vi "CSC_InitCableLocation.vi"(8 "error in (no error)":errorcluster, 11 "C-Alex in":refnum<class "CableSerialChain.lvclass">) -> (0 "error out":errorcluster, 3 "C-Alex out":refnum<class "CableSerialChain.lvclass">)   [LabVIEW 2014]
uses:
  Body/PointOnBody.ctl
  Body/Bodies.lvclass
  Cable.ctl
  CableSerialChain.lvclass
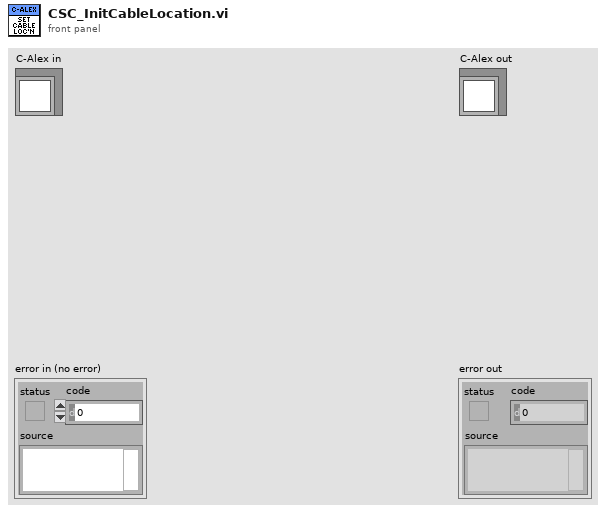
[diagram p1: front panel]
types:
  T1 = typedef "CableSerialChain.lvclass/Cable.ctl" = cluster{"RoutingPtsInLegCoSys":T2[], "Cable ID":i32}
  T2 = typedef "Bodies.lvclass/PointOnBody.ctl" = cluster{"Coord4":dbl[], "ID":i32}
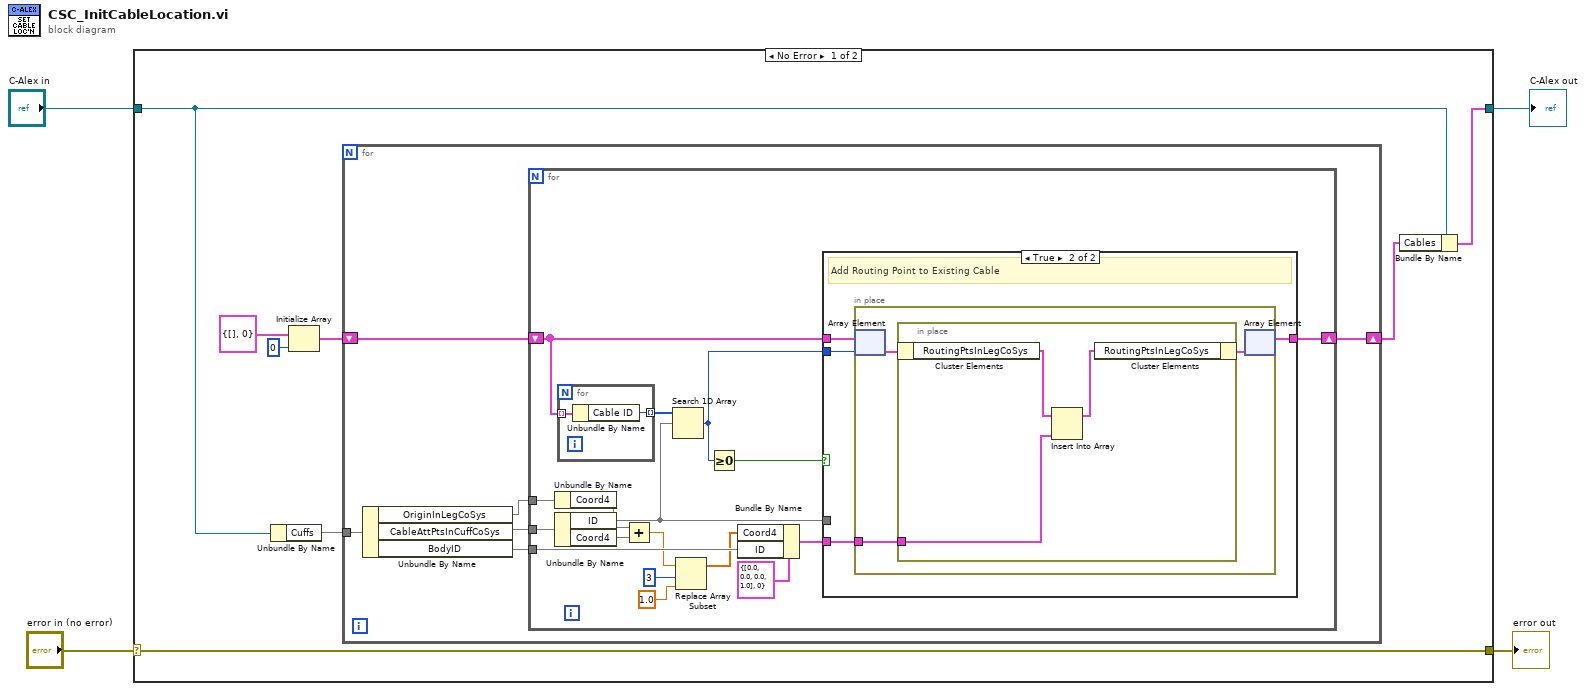
[diagram p0: block diagram]
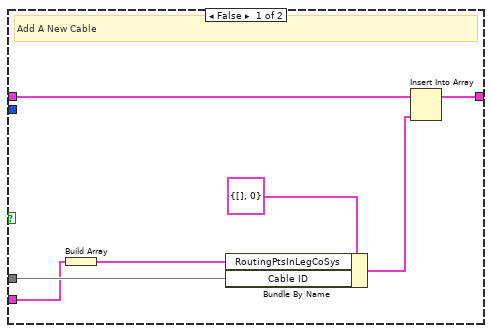
[diagram p2: hidden frame]
diagram:
  n1 = case shown="No Error" "error in (no error)" {
    selector: "error in (no error)" -> [w12 w56]
    tunnel: [w12 w56] -> w3
    tunnel: [w5 w55] -> w1
    tunnel: "C-Alex in" -> [w10 w55]
    frame No Error {
      n2 = Unbundle By Name(w10) -> ("Cuffs"=w11)
      n3 = Initialize Array(T1 {"RoutingPtsInLegCoSys"=[], "Cable ID"=0} ("Cable"), 0 ("dimension size")) -> (w9:T1[])
      n4 = for {
        tunnel: w11 -> [w18]
        shift-right: [w14] -> w6
        shift-left: w9 -> [w15]
        n5 = Unbundle By Name(w18) -> ("OriginInLegCoSys"=w13, "CableAttPtsInCuffCoSys"=w17, "BodyID"=w16)
        n6 = for {
          tunnel: w17 -> [w35]
          tunnel: w16 -> [w33]
          shift-right: [w28] -> w14
          shift-left: w15 -> [w26]
          tunnel: w13 -> [w25]
          n7 = Unbundle By Name(w25) -> ("Coord4"=w23)
          n8 = Unbundle By Name(w35) -> ("ID"=w27, "Coord4"=w24)
          n9 = for {
            tunnel: w26 -> [w54] mode=indexing
            tunnel: [w53] -> w32 mode=indexing
            n10 = Unbundle By Name(w54) -> ("Cable ID"=w53:i32)
          }
          n11 = Add(x=w23, y=w24) -> (x+y=w22:dbl)
          n12 = Search 1D Array(1D array=w32, element=w27) -> (index of element=w30:i32)  [unwired: 1 in]
          n13 = Replace Array Subset(array=w22, new element=1.0 ("new element/subarray"), index=3) -> (w21:dbl[])
          n14 = Greater Or Equal To 0?(x=w30) -> (x >= 0?=w31:bool)
          n15 = Bundle By Name(cluster=T2 {"Coord4"=[0.0, 0.0, 0.0, 1.0], "ID"=0} ("Point"), "Coord4"=w21, "ID"=w33) -> (w29:T2)
          n16 = case shown="True" w31 {
            tunnel: w30 -> [_ w45]
            tunnel: w26 -> [w42 w46]
            tunnel: w29 -> [w37 w43]
            tunnel: [w39 w44] -> w28
            tunnel: w27 -> [w40 _]
            frame False {
              # "Add A New Cable"
              n17 = Build Array(w37) -> (w36:T2[])
              n18 = Bundle By Name(cluster=T1 {"RoutingPtsInLegCoSys"=[], "Cable ID"=0} ("Cable"), "RoutingPtsInLegCoSys"=w36, "Cable ID"=w40) -> (w38:T1)
              n19 = Insert Into Array(array=w42, new element=w38) -> (w39:T1[])  [unwired: 1 in]
            }
            frame True {
              # "Add Routing Point to Existing Cable"
              n20 = in-place {
                in-place-border: w43 -> [w48]
                n21 = in-place-array #1(w46, w45) -> (w49:T1)
                n22 = in-place {
                  in-place-border: w48 -> [w51]
                  n23 = in-place-cluster #2(w49) -> ("RoutingPtsInLegCoSys"=w52:T2[])
                  n24 = Insert Into Array(array=w52, new element=w51) -> (w50:T2[])  [unwired: 1 in]
                  n25 = in-place-cluster #2("RoutingPtsInLegCoSys"=w50) -> (w47:T1)
                }
                n26 = in-place-array #1(w47) -> (w44:T1[])  [unwired: 1 out]
              }
            }
          }
        }
      }
      n27 = Bundle By Name(cluster=w10, "Cables"=w6) -> (w5:cluster{})
    }
    frame Error {
    }
  }
  "error out" <- w3
  "C-Alex out" <- w1
